vi "GetAllVIFileName.vi"() -> (1 "去掉后缀":string[](array[string]), 2 "VI文件名":string[](array[string]), 3 "路径输出":path)   [LabVIEW 2018]
panel:
  out "error out":errorcluster caption="错误输出"
  in  "error in (no error)":errorcluster caption="错误输入（无错误）"
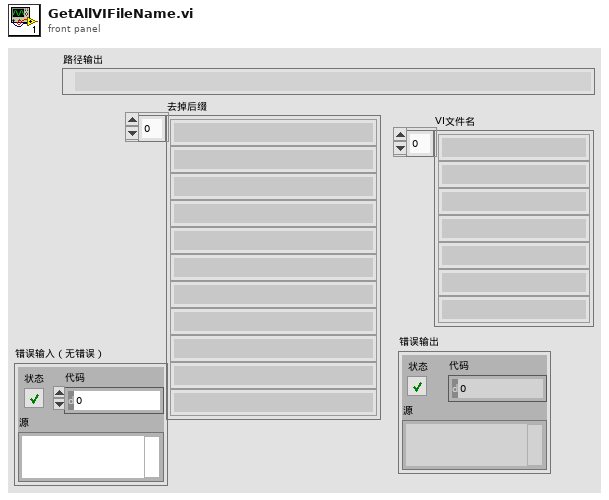
[diagram p1: front panel]
types:
  T1 = enum32{"invalid app kind", "Development System", "Run Time System", "Student Edition", "Embedded LabVIEW", "Evaluation", "Custom"}
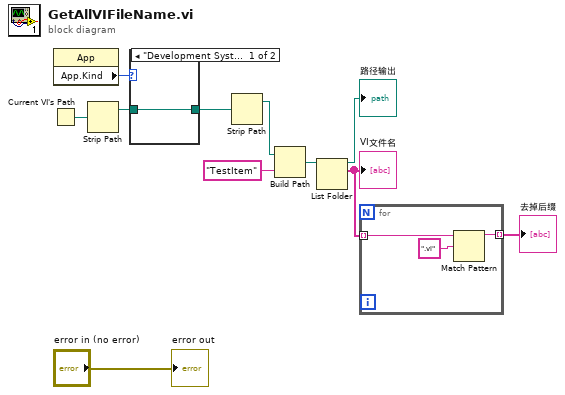
[diagram p0: block diagram]
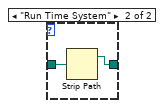
[diagram p2: hidden frame]
diagram:
  n1 = Current VI's Path() -> (path=w10:path)
  n2 = property class="App"() -> ("App.Kind"=w9:T1)  [unwired: 2 in, 2 out]
  n3 = Strip Path(path=w10) -> (stripped path=w11:path)  [unwired: 1 out]
  n4 = case shown="\"Development System\", 默认" w9 {
    tunnel: w11 -> [w12 w14]
    tunnel: [w12 w13] -> w8
    frame "Development System", Default {
    }
    frame "Run Time System" {
      n5 = Strip Path(path=w14) -> (stripped path=w13:path)  [unwired: 1 out]
    }
  }
  n6 = Strip Path(path=w8) -> (stripped path=w6:path)  [unwired: 1 out]
  n7 = Build Path(base path=w6, name or relative path="TestItem" ("名称或相对路径")) -> (appended path=w2:path)
  n8 = List Folder(path=w2) -> (path out=→"路径输出":path, filenames=w4:string[])  [unwired: 3 in, 2 out]
  "VI文件名" <- w4
  n9 = for {
    tunnel: w4 -> [w17] mode=indexing
    tunnel: [w15] -> w3 mode=indexing
    n10 = Match Pattern(string=w17, regular expression=".vi" ("正则表达式")) -> (before substring=w15:string)  [unwired: 1 in, 3 out]
  }
  "去掉后缀" <- w3
  "error out" <- "error in (no error)"
